vi "Dequeue for model.vi"(0 "timeout in ms (-1, no timeout)":i32=-1, 7 "State to run on timeout (Timeout)":string, 11 "error in (no error)":errorcluster, 12 "Fiber Auto Collimation state data in":refnum<class "Fiber Auto Collimation state data.lvclass">) -> (2 "Next state if error":string, 4 "Data":variant, 8 "Enqueued state":string, 14 "Fiber Auto Collimation state data out":refnum<class "Fiber Auto Collimation state data.lvclass">, 15 "error out":errorcluster)   [LabVIEW 2018]
doc: "This VI:\n1. Gets the model queue reference\n2. Checks if the queue is empty. If so, sets the \"Model case running\" value to \"Idle\".\n3. Waits for a queue object (or a timeout, if wired)\n4. Unpacks the queue object data\n5. Set the \"Model case running\" value to the name of the enqueued state.\n6. Passes out the unpacked queue elements (state, data, next state on error)."
uses:
  State data/Fiber Auto Collimation state data.lvclass
  State data/Fiber Auto Collimation state data.lvclass/Fiber Auto Collimation state data.ctl
  <vilib>/Utility/error.llb/Clear Errors.vi
  State data/Add Changed data.vi
  <userlib>/nLight Error Handling/Log any errors.vi
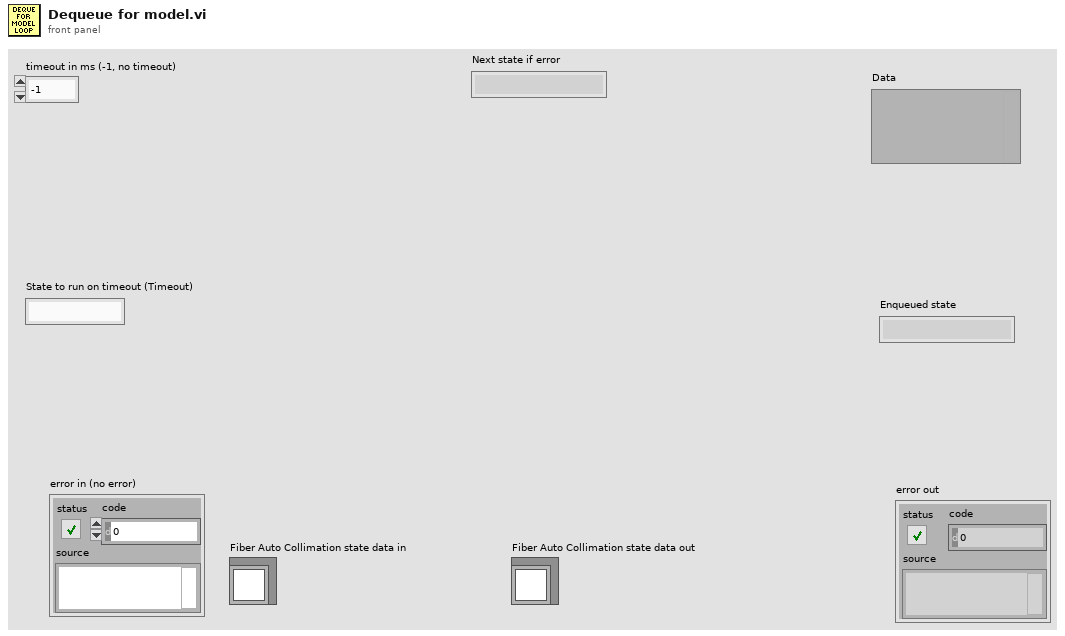
[diagram p1: front panel]
types:
  T1 = typedef "Model queue data.ctl" = cluster{"State":string, "Data":variant, "Next state if error":string}
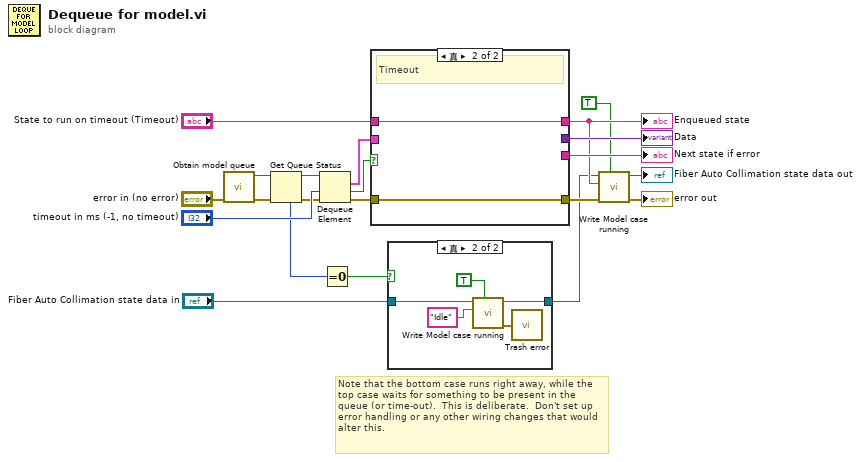
[diagram p0: block diagram]
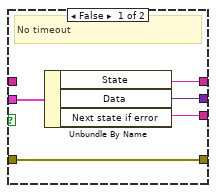
[diagram p3: hidden frame]
diagram:
  # "Note that the bottom case runs right away, while the top case waits for something to be present in the queue (or time-out).  This is deliberate.  Don't set up error handling or any other wiring changes that would alter this."
  n1 = call "Obtain model queue.vi"("error in (no error)"="error in (no error)") -> ("error out"=w20:errorcluster, "Model loop queue"=w11:refnum<queue>)  [unwired: 9 in]
  n2 = Get Queue Status(queue=w11, error in (no error)=w20) -> (queue out=w10:refnum<queue>, error out=w12:errorcluster, # elements in queue=w9:i32)  [unwired: 1 in, 5 out]
  n3 = Dequeue Element(queue=w10, timeout in ms (-1)="timeout in ms (-1, no timeout)", error in (no error)=w12) -> (element=w16:T1, timed out?=w17:bool, error out=w18:errorcluster)  [unwired: 1 out]
  n4 = Equal To 0?(x=w9) -> (x = 0?=w7:bool)
  n5 = case shown="真" w17 {
    tunnel: w18 -> [w23 w28]
    tunnel: w16 -> [w22 _]
    tunnel: "State to run on timeout (Timeout)" -> [_ w27]
    tunnel: [w26 w27] -> w3
    tunnel: [w25 _] -> w14
    tunnel: [w24 _] -> w13
    tunnel: [w23 w28] -> w6
    frame False {
      # "No timeout"
      n6 = Unbundle By Name(w22) -> ("State"=w26:string, "Data"=w25:variant, "Next state if error"=w24:string)
    }
    frame True {
      # "Timeout"
    }
  }
  "Next state if error" <- w13
  "Data" <- w14
  "Enqueued state" <- w3
  n7 = case shown="真" w7 {
    tunnel: "Fiber Auto Collimation state data in" -> [w29 w34]
    tunnel: [w29 w31] -> w1
    frame False {
    }
    frame True {
      n8 = call "Write Model case running.vi"("Send any changes now? (F)"=TRUE, "Model case running"="Idle" ("Controller case running"), "Fiber Auto Collimation state data in"=w34) -> ("error out"=w30:errorcluster, "Fiber Auto Collimation state data out"=w31:refnum<class "Fiber Auto Collimation state data.lvclass">)  [unwired: 7 in]
      n9 = call <userlib>:"Trash error.vi"("error in"=w30) -> ()  [unwired: 15 in]
    }
  }
  n10 = call "Write Model case running.vi"("Send any changes now? (F)"=TRUE, "error in (no error)"=w6, "Model case running"=w3, "Fiber Auto Collimation state data in"=w1) -> ("error out"=→"error out":errorcluster, "Fiber Auto Collimation state data out"=→"Fiber Auto Collimation state data out":refnum<class "Fiber Auto Collimation state data.lvclass">)  [unwired: 6 in]
